vi "Configure Advanced Trigger [AT].vi"(7 "Trigger Slope (Positive)":i32(ring) caption="trigger slope (Positive)" items=["Positive", "Negative", "Either"], 8 "error in (no error)":errorcluster, 9 "Trigger Source (None)":string(combo) caption="trigger source (None)", 10 "Channel Name (\"\")":string="CHANNEL1" caption="channel name (\"CHANNEL1\")", 11 "CS++Fgen in":refnum<class "CS++Fgen.lvclass">) -> (0 "error out":errorcluster, 3 "CS++Fgen out":refnum<class "CS++Fgen.lvclass">)   [LabVIEW 2013, in "CS++Fgen.lvlib" / "CS++Fgen.lvclass"]
doc: "This VI configures the properties that control the function generator's advance trigger. These properties are the advance trigger source and slope.\n\nAn advance trigger advances generation to the end of the current waveform, where generation proceeds according to the current configuration.\n\nNote:\n\n(1) This VI is part of the IviFgenAdvanceTrigger [AT] extension group."
uses:
  CS++Fgen.lvclass
  CSPP_Core/Classes/CS++ProcessVariables/ProcessVariable/PV.lvclass
  PV-Enum-n.ctl
  CSPP_Core/Classes/CS++ProcessVariables/ProcessVariable/PV.lvclass/PV.ctl
  CS++Fgen.lvclass/CS++Fgen.ctl
  CSPP_Core/Classes/CS++ProcessVariables/PVConnection/PVConnection.lvclass
  CSPP_Core/Classes/CS++ProcessVariables/ProcessVariable/Write Data.vi
  CSPP_Core/Classes/CS++ProcessVariables/ProcessVariable/Write Timestamp.vi
  CSPP_Core/Classes/CS++ProcessVariables/ProcessVariable/Write Quality.vi
  CSPP_Core/Classes/CS++ProcessVariables/ProcessVariable/Write status.vi
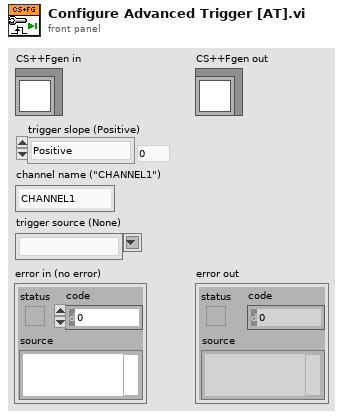
[diagram p1: front panel]
types:
  T1 = typedef "CS++Fgen.lvlib/CS++Fgen.lvclass/PV-Enum-n.ctl" = enum16{"Amplitude", "Arb-Frequency", "DCOffset", "Frequency", "OutputImpedance", "StartPhase", "AdvancedTriggerSlope", "AM-Source", "BurstCount", "FM-Source", "OperationMode", "ResumeTriggerSlope", "StartTriggerSlope", "StopTriggerSlope", "Waveform", "AM-Enabled", "ChannelEnabled", "FM-Enabled", "AdvancedTriggerSource", "ResumeTriggerSource", "StartTriggerSource", "StopTriggerSource", "TriggerSource"}
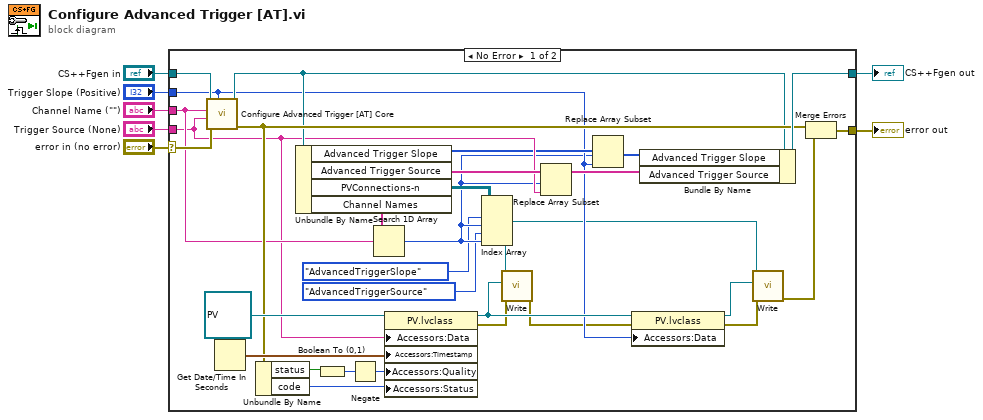
[diagram p0: block diagram]
diagram:
  n1 = case shown="No Error" "error in (no error)" {
    selector: "error in (no error)" -> [w38 w41]
    tunnel: [w26 w41] -> w6
    tunnel: [w25 w40] -> w4
    tunnel: "CS++Fgen in" -> [w39 w40]
    tunnel: "Trigger Slope (Positive)" -> [w17 _]
    tunnel: "Channel Name (\"\")" -> [w22 _]
    tunnel: "Trigger Source (None)" -> [w21 _]
    frame No Error {
      n2 = call-dynamic "Configure Advanced Trigger [AT] Core.vi"("Trigger Slope (Positive)"=w17, "error in (no error)"=w38, "Trigger Source (None)"=w21, "Channel Name (\"\")"=w22, "CS++Fgen in"=w39) -> ("error out"=w24:errorcluster, "CS++Fgen out"=w23:refnum<class "CS++Fgen.lvclass">)  [unwired: 5 in]
      n3 = Get Date/Time In Seconds() -> (seconds since 1Jan1904=w37:timestamp)
      n4 = Unbundle By Name(w24) -> ("status"=w32:bool, "code"=w30:i32)
      n5 = Unbundle By Name(w23) -> ("Advanced Trigger Slope"=w20:i32[], "Advanced Trigger Source"=w28:string[], "PVConnections-n"=w34:refnum<class "PVConnection.lvclass">[][], "Channel Names"=w35:string[])
      n6 = Boolean To (0,1)(Boolean=w32) -> (0, 1=w31:i16)
      n7 = Negate(x=w31) -> (-x=w29:i16)
      n8 = Search 1D Array(1D array=w35, element=w22) -> (index of element=w11:i32)  [unwired: 1 in]
      n9 = property class="PV.lvclass"(reference=refnum<class "PV.lvclass"> refnum ("PV"), "Accessors:Data"=w21, "Accessors:Timestamp"=w37, "Accessors:Quality"=w29, "Accessors:Status"=w30) -> (reference out=w18:refnum<class "PV.lvclass">, error out=w13:errorcluster)  [unwired: 1 in]
      n10 = Index Array(array=w34, index (row) #1=PV-Enum-n."AdvancedTriggerSlope" ("PV-Enum-n"), index (col) #1=w11, index (row) #2=PV-Enum-n."AdvancedTriggerSource" ("PV-Enum-n"), index (col) #2=w11) -> (element #1=w8:refnum<class "PVConnection.lvclass">, element #2=w33:refnum<class "PVConnection.lvclass">)
      n11 = call-dynamic "Write.vi"("error in (no error)"=w13, "PV"=w18, "PVConnection in"=w33) -> ("error out"=w12:errorcluster)  [unwired: 7 in, 1 out]
      n12 = Replace Array Subset(array=w28, new element=w21, index=w11) -> (w27:string[])
      n13 = Replace Array Subset(array=w20, new element=w17, index=w11) -> (w19:i32[])
      n14 = property class="PV.lvclass"(reference=w18, error in=w12, "Accessors:Data"=w17) -> (reference out=w15:refnum<class "PV.lvclass">, error out=w14:errorcluster)
      n15 = Bundle By Name(cluster=w23, "Advanced Trigger Slope"=w19, "Advanced Trigger Source"=w27) -> (w25:refnum<class "CS++Fgen.lvclass">)
      n16 = call-dynamic "Write.vi"("error in (no error)"=w14, "PV"=w15, "PVConnection in"=w8) -> ("error out"=w16:errorcluster)  [unwired: 7 in, 1 out]
      n17 = Merge Errors(w24, w16) -> (w26:errorcluster)
    }
    frame Error {
    }
  }
  "error out" <- w6
  "CS++Fgen out" <- w4
